vi "Go to Position.vi"(0 "X (mm)":sgl, 1 "Speed (2000 mm/min)":sgl=2000.0, 2 "Overwright speed? (F)":bool, 5 "Y (mm)":sgl, 7 "Z (mm)":sgl, 9 "Wait for finish? (T)":bool=TRUE, 11 "error in (no error)":errorcluster) -> (15 "error out":errorcluster)   [LabVIEW 2024, in "GRBL 1.1.lvlib"]
doc: "This vi send the command to go to next position."
uses:
  GRBL 1.1.lvlib
  Status.ctl
panel:
  in  "WPos":bool
  out "Data read":string
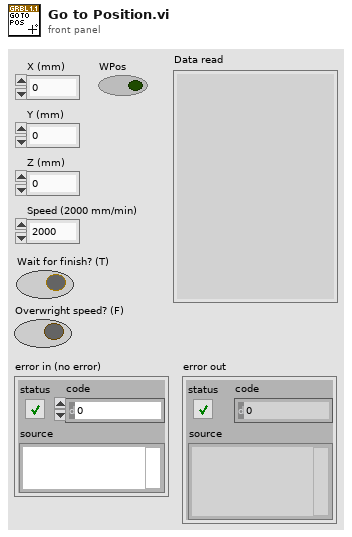
[diagram p1: front panel]
types:
  T1 = typedef "GRBL 1.1.lvlib/Status.ctl" = enum16{"", "Alarm", "Idle", "Run", "Home"}
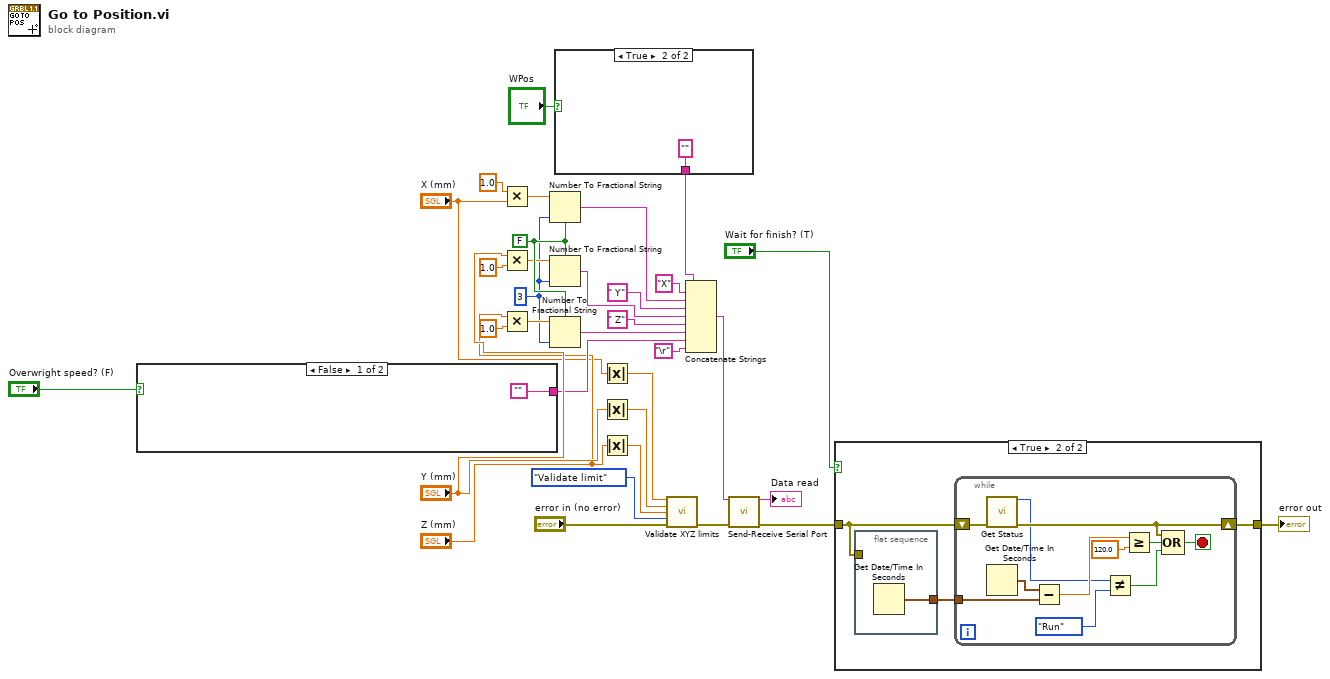
[diagram p0: block diagram]
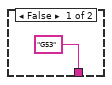
[diagram p2: hidden frame]
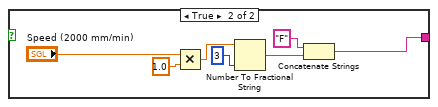
[diagram p3: hidden frame]
diagram:
  w10 = i16 3 ("precision (6)")
  w24 = FALSE ("use system decimal point (T)")
  n1 = case shown="False" "Overwright speed? (F)" {
    tunnel: ["" w36] -> w9
    frame False {
    }
    frame True {
      n2 = Multiply(x="Speed (2000 mm/min)", y=sgl 1.0) -> (x*y=w41:sgl)
      n3 = Number To Fractional String(number=w41, precision (6)=i16 3) -> (F-format string=w37:string)  [unwired: 2 in]
      n4 = Concatenate Strings("F" ("string"), w37) -> (w36:string)
    }
  }
  n5 = Multiply(x=sgl 1.0 ("y"), y="X (mm)") -> (x*y=w17:sgl)
  n6 = Multiply(x="Y (mm)", y=sgl 1.0) -> (x*y=w15:sgl)
  n7 = Multiply(x="Z (mm)", y=sgl 1.0) -> (x*y=w13:sgl)
  n8 = Number To Fractional String(use system decimal point (T)=w24, number=w17, precision (6)=w10) -> (F-format string=w28:string)  [unwired: 1 in]
  n9 = Number To Fractional String(use system decimal point (T)=w24, number=w15, precision (6)=w10) -> (F-format string=w27:string)  [unwired: 1 in]
  n10 = Number To Fractional String(use system decimal point (T)=w24, number=w13, precision (6)=w10) -> (F-format string=w26:string)  [unwired: 1 in]
  n11 = case shown="True" "WPos" {
    tunnel: ["G53" ""] -> w1
    frame False {
    }
    frame True {
    }
  }
  n12 = Absolute Value(x="X (mm)") -> (abs(x)=w5:sgl)
  n13 = Absolute Value(x="Y (mm)") -> (abs(x)=w4:sgl)
  n14 = Absolute Value(x="Z (mm)") -> (abs(x)=w3:sgl)
  n15 = call "Validate XYZ limits.vi"("X"=w5, "Y"=w4, "Z"=w3, "Action"=enum16{"Set Limit", "Validate limit"}."Validate limit", "error in (no error)"="error in (no error)") -> ("error out"=w23:errorcluster)  [unwired: 9 in, 1 out]
  n16 = Concatenate Strings(w1, "X", w28, " Y" ("string"), w27, " Z" ("string"), w26, w9, "\r") -> (w33:string)
  n17 = call "Send-Receive Serial Port.vi"("Data to write"=w33, "error in (no error)"=w23) -> ("Data read"=→"Data read":string, "error out"=w18:errorcluster)  [unwired: 12 in]
  n18 = case shown="True" "Wait for finish? (T)" {
    tunnel: [w44 w47] -> w20
    tunnel: w18 -> [w44 w45]
    frame False {
    }
    frame True {
      n19 = flat-sequence {
        tunnel: [w48] -> w46
        tunnel: w45 -> [_]
        frame #0 {
          n20 = Get Date/Time In Seconds() -> (seconds since 1Jan1904=w48:timestamp)
        }
      }
      n21 = while {
        shift-right: [w52] -> w47
        shift-left: w45 -> [w59]
        tunnel: w46 -> [w56]
        stop <- w58 stop-if-true
        n22 = call "Get Status.vi"("error in (no error)"=w59) -> ("Status"=w51:T1, "error out"=w52:errorcluster)  [unwired: 10 in, 3 out]
        n23 = Get Date/Time In Seconds() -> (seconds since 1Jan1904=w57:timestamp)
        n24 = Subtract(x=w57, y=w56) -> (x-y=w55:dbl)
        n25 = Not Equal?(x=w51, y=Status."Run") -> (x != y?=w49:bool)
        n26 = Greater Or Equal?(x=w55, y=120.0) -> (x >= y?=w53:bool)
        n27 = Compound Arithmetic op=OR(w52, w53, w49) -> (w58:bool)
      }
    }
  }
  "error out" <- w20
